vi "SL_ValueDialog.vi"(10 "Value":string, 11 "Title":string) -> (1 "replace?":bool, 2 "Value out":string)   [LabVIEW 2019]
panel:
  in  "Cancel Button":bool
  in  "OK Button":bool
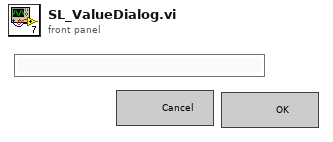
[diagram p1: front panel]
types:
  T1 = enum8{"Enabled", "Disabled", "Disabled and Grayed Out"}
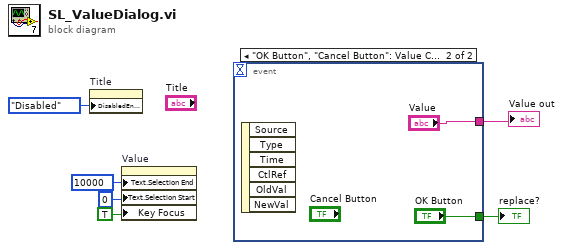
[diagram p0: block diagram]
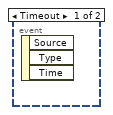
[diagram p2: hidden frame]
diagram:
  n1 = property on="Title" class="Str"("DisabledEnum"=T1."Disabled" ("Disabled")) -> ()  [unwired: 2 in, 2 out]
  n2 = property on="Value" class="Str"("Text.Selection End"=u32 10000 ("Text.Selection:End"), "Text.Selection Start"=u32 0 ("Text.Selection:Start"), "Key Focus"=TRUE) -> ()  [unwired: 2 in, 2 out]
  n3 = event shown="[1] \"OK Button\", \"Cancel Button\": Value Change" {
    selector: _ -> [_ _]
    dyn-events: _ -> [_ _]
    timeout: _ -> [_ _]
    tunnel: [_ "OK Button"] -> w5
    tunnel: [_ "Value"] -> w4
    event Timeout {
      n4 = event-data() -> ()  [unwired: 1 in, 3 out]
    }
    event "OK Button", "Cancel Button": Value Change {
      n5 = event-data() -> ()  [unwired: 1 in, 6 out]
    }
  }
  "Value out" <- w4
  "replace?" <- w5
